vi "Set TC Type.vi"(8 "error in (no error)":errorcluster, 10 "Thermocouple Type (4: K)":u32(ring)=4 items=["B", "C", "E", "J", "K", "L:Jdin", "N", "R", "S", "T", "U:Tdin", "X", "Y", "Z"], 11 "VISA resource name":refnum<visa-resource-name>) -> (0 "error out":errorcluster, 3 "VISA resource name out":refnum<visa-resource-name>)   [LabVIEW 2014, in "Fluke 5XXX Series Multicalibrators.lvlib"]
doc: "This VI sets the Thermocouple (TC) temperature sensor type. The TC type is used when the output is set to a temperature value with the FL5XCAL Get Output Values.vi and the temperature sensor type is set to TC with the FL5XCAL Set Temp Sensor Type.vi . When the thermocouple type is changed while simulating a temperature output, the temperature is changed to 0 °C. Once set, the Calibrator retains the TC type until power off or reset.\n\nNote:\n\nThis VI is available only for instrument models 5500A and 5520A."
uses:
  Fluke 5XXX Series Multicalibrators.lvlib
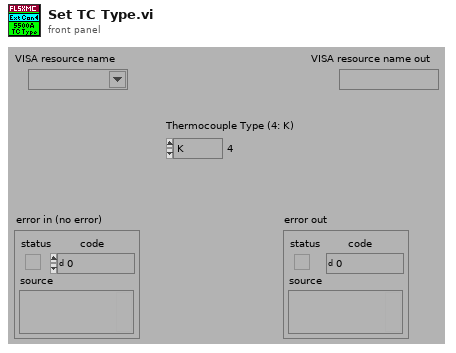
[diagram p1: front panel]
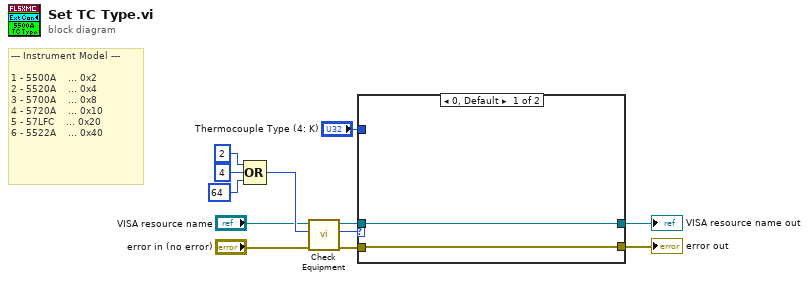
[diagram p0: block diagram]
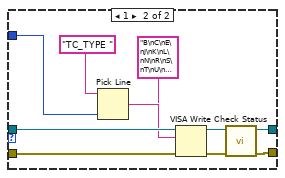
[diagram p2: hidden frame]
diagram:
  # "--- Instrument Model ---\n\n1 - 5500A    ... 0x2\n2 - 5520A    ... 0x4\n3 - 5700A    ... 0x8\n4 - 5720A    ... 0x10\n5 - 57LFC    ... 0x20\n6 - 5522A    ... 0x40"
  n1 = Compound Arithmetic op=OR(2 ("Numeric"), 4 ("Numeric"), 64 ("Numeric")) -> (w9:i32)
  n2 = call "Check Equipment.vi"("error in (no error)"="error in (no error)", "Bit Mask"=w9, "VISA resource name"="VISA resource name") -> ("error out"=w12:errorcluster, "Present?"=w11:u32, "VISA resource name out"=w10:refnum<visa-resource-name>)  [unwired: 6 in]
  n3 = case shown="0, Default" w11 {
    tunnel: "Thermocouple Type (4: K)" -> [_ w20]
    tunnel: [w13 w16] -> w2
    tunnel: w12 -> [w14 w23]
    tunnel: w10 -> [w13 w22]
    tunnel: [w14 w19] -> w3
    frame 0, Default {
    }
    frame 1 {
      n4 = Pick Line(string ("")="TC_TYPE " ("Reset Command"), multi-line string="B\nC\nE\nJ\nK\nL\nN\nR\nS\nT\nU\nX\nY\nZ", line index=w20) -> (output string=w21:string)
      n5 = VISA Write(VISA resource name=w22, write buffer=w21, error in (no error)=w23) -> (VISA resource name out=w17:refnum<visa-resource-name>, error out=w18:errorcluster)  [unwired: 1 out]
      n6 = call "Check Status.vi"("VISA resource name"=w17, "error in (no error)"=w18) -> ("VISA resource name out"=w16:refnum<visa-resource-name>, "error out"=w19:errorcluster)  [unwired: 12 in]
    }
  }
  "VISA resource name out" <- w2
  "error out" <- w3
